vi "Waiting_Sweep_Status.vi"(8 "error in (no error)":errorcluster, 9 "status":i32(ring) items=["Standby", "Running", "Pausing", "WaitingforTrigger", "Returning"], 10 "Wait time(msec)":i32, 11 ".NET Reference in":refnum<k24>) -> (0 "error out":errorcluster, 3 "Reference out":refnum<k24>)   [LabVIEW 2017]
uses:
  C:/Users/Ssantec_Test/Documents/Instrument_DLL_Sample_Labview_20220902_Ver1.2.2/DLL/x86/InstrumentDLL.dll
  DLL/x86/InstrumentDLL.dll
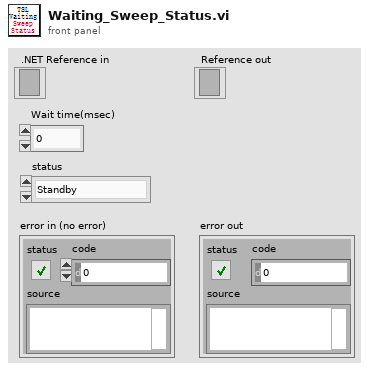
[diagram p1: front panel]
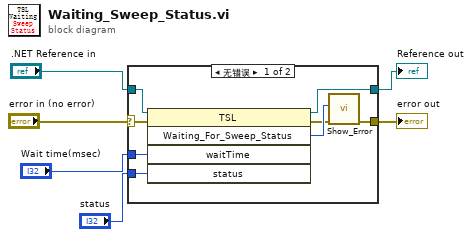
[diagram p0: block diagram]
diagram:
  n1 = case shown="无错误" "error in (no error)" {
    selector: "error in (no error)" -> [w7 w15]
    tunnel: "Wait time(msec)" -> [w14 _]
    tunnel: "status" -> [w13 _]
    tunnel: ".NET Reference in" -> [w12 w16]
    tunnel: [w11 w16] -> w4
    tunnel: [w8 w15] -> w3
    frame No Error {
      n2 = invoke on="调用节点" class="TSL" method="Waiting_For_Sweep_Status"(reference=w12, error in=w7, "waitTime"=w14, "status"=w13) -> (reference out=w11:refnum<k24>, error out=w9:errorcluster, "Waiting_For_Sweep_Status"=w10:i32)  [unwired: 1 in, 2 out]
      n3 = call "Show_Error.vi"("error in (no error)"=w9, "Error"=w10) -> ("error out"=w8:errorcluster)  [unwired: 9 in]
    }
    frame Error {
    }
  }
  "Reference out" <- w4
  "error out" <- w3
